vi "Set Owning Object.vi"(7 "Set Absolute":bool, 8 "error in (no error)":errorcluster, 9 "Absolute Positions":T1[](array[typedef]), 10 "All Controls In":refnum<vi>[](array[refnum]), 11 "Owner Object":refnum<vi>) -> (0 "error out":errorcluster, 1 "Positions":T1[](array[typedef]), 3 "All Controls Out":refnum<vi>[](array[refnum]))   [LabVIEW 2013]
uses:
  <vilib>/Utility/miscctls.llb/LVPositionTypeDef.ctl
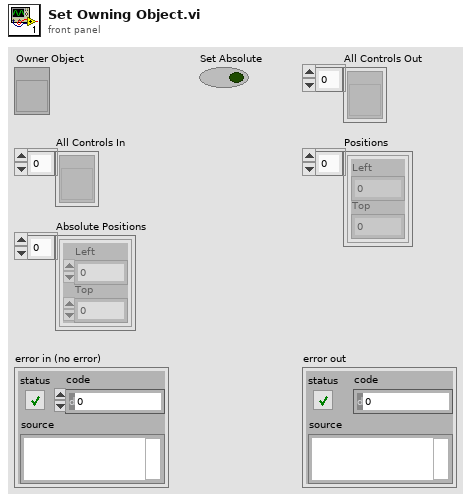
[diagram p1: front panel]
types:
  T1 = typedef "LVPositionTypeDef.ctl" = cluster{"Left":i32, "Top":i32}
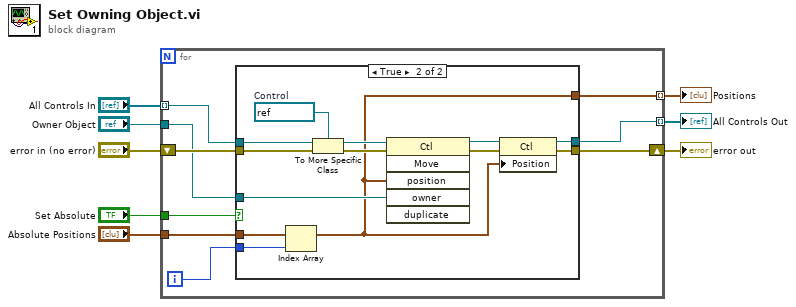
[diagram p0: block diagram]
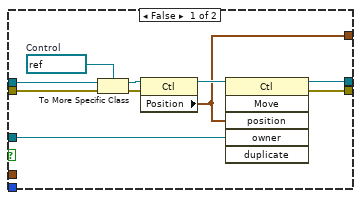
[diagram p2: hidden frame]
diagram:
  n1 = for {
    tunnel: "All Controls In" -> [w13] mode=indexing
    tunnel: "Owner Object" -> [w15]
    tunnel: [w14] -> w8 mode=indexing
    shift-right: [w16] -> w6
    shift-left: "error in (no error)" -> [w17]
    tunnel: "Absolute Positions" -> [w11]
    tunnel: [w12] -> w2 mode=indexing
    tunnel: "Set Absolute" -> [w10]
    i -> [w9]
    n2 = case shown="True" w10 {
      tunnel: w17 -> [w27 w40]
      tunnel: [w26 w31] -> w16
      tunnel: w15 -> [w25 w39]
      tunnel: [w24 w29] -> w14
      tunnel: w13 -> [w22 w36]
      tunnel: [w18 w28] -> w12
      tunnel: w11 -> [_ w33]
      tunnel: w9 -> [_ w32]
      frame False {
        w21 = refnum<vi> refnum  # Control
        n3 = To More Specific Class(target class=w21, reference=w22, error in=w27) -> (specific class reference=w20:refnum<vi>, error out=w23:errorcluster)
        n4 = property class="Ctl"(reference=w20, error in=w23) -> (reference out=w19:refnum<vi>, "Position"=w18:T1)  [unwired: 1 out]
        n5 = invoke class="Ctl" method="Move"(reference=w19, "position"=w18, "owner"=w25) -> (reference out=w24:refnum<vi>, error out=w26:errorcluster)  [unwired: 3 in, 4 out]
      }
      frame True {
        w34 = refnum<vi> refnum  # Control
        n6 = Index Array(array=w33, index=w32) -> (element=w28:T1)
        n7 = To More Specific Class(target class=w34, reference=w36, error in=w40) -> (specific class reference=w35:refnum<vi>, error out=w37:errorcluster)
        n8 = invoke class="Ctl" method="Move"(reference=w35, error in=w37, "position"=w28, "owner"=w39) -> (reference out=w30:refnum<vi>, error out=w38:errorcluster)  [unwired: 2 in, 4 out]
        n9 = property class="Ctl"(reference=w30, error in=w38, "Position"=w28) -> (reference out=w29:refnum<vi>, error out=w31:errorcluster)
      }
    }
  }
  "All Controls Out" <- w8
  "error out" <- w6
  "Positions" <- w2
